vi "Actor Core.vi"(8 "error in":errorcluster, 11 "Settings Actor in":refnum<class "Settings Actor.lvclass">) -> (0 "error out":errorcluster, 3 "Actor out":refnum<class "Actor.lvclass">)   [LabVIEW 2021, in "Settings Module.lvlib" / "Settings Actor.lvclass"]
doc: "The user interface for this panel.\n\n----\nPlease see the following web address for additional documentation and tutorial information:\nhttp://www.mooregoodideas.com/mgi-panel-manager/\n\nAuthor: Derek Trepanier\n\nCopyright (c) 2018, Moore Good Ideas, Inc.\n\nAll rights reserved.\n\nRedistribution and use in source and binary forms, with or without modification, are permitted provided that the following conditions are met:\n\n * Redistributions of source code must retain the above copyright notice, this list of conditions and the following disclaimer.\n * Redistributions in binary form must reproduce the above copyright notice, this list of conditions and the following disclaimer in the documentation and/or other materials provided with the distribution.\n * Neither the name of Moore Good Ideas, Inc. nor the names of its contributors may be used to endorse or promote products derived from this software without specific prior written permission.\n\nTHIS SOFTWARE IS PROVIDED BY THE COPYRIGHT HOLDERS AND CONTRIBUTORS \"AS IS\" AND ANY EXPRESS OR IMPLIED WARRANTIES, INCLUDING, BUT NOT LIMITED TO, THE IMPLIED WARRANTIES OF MERCHANTABILITY AND FITNESS FOR A PARTICULAR PURPOSE ARE DISCLAIMED. IN NO EVENT SHALL THE COPYRIGHT OWNER OR CONTRIBUTORS BE LIABLE FOR ANY DIRECT, INDIRECT, INCIDENTAL, SPECIAL, EXEMPLARY, OR CONSEQUENTIAL DAMAGES (INCLUDING, BUT NOT LIMITED TO, PROCUREMENT OF SUBSTITUTE GOODS OR SERVICES; LOSS OF USE, DATA, OR PROFITS; OR BUSINESS INTERRUPTION) HOWEVER CAUSED AND ON ANY THEORY OF LIABILITY, WHETHER IN CONTRACT, STRICT LIABILITY, OR TORT (INCLUDING NEGLIGENCE OR OTHERWISE) ARISING IN ANY WAY OUT OF THE USE OF THIS SOFTWARE, EVEN IF ADVISED OF THE POSSIBILITY OF SUCH DAMAGE."
uses:
  Settings Actor.lvclass
  C:/Program Files (x86)/National Instruments/LabVIEW 2021/vi.lib/MGI/Panel Manager/Panel Actor/Panel Actor/Panel Actor.lvclass
  <vilib>/ActorFramework/Actor/Actor.lvclass
  <vilib>/ActorFramework/Message Enqueuer/Message Enqueuer.lvclass/Message Enqueuer.ctl
  Appearance Actor/Appearance Actor/Typedefs/User Event-Panel Resize-Data--cluster.ctl
  <vilib>/Utility/miscctls.llb/LVRectTypeDef.ctl
  <vilib>/event_ctls.llb/sizeaction.ctl
  <vilib>/event_ctls.llb/panelstate.ctl
  Appearance Actor/Appearance Actor Messages/User Event-Panel Resize Msg/User Event-Panel Resize Msg.lvclass/User Event-Panel Resize Msg.ctl
  <vilib>/ActorFramework/Message Enqueuer/Enqueue.vi
  <vilib>/ActorFramework/Stop Msg/Stop Msg.lvclass
  C:/Program Files (x86)/National Instruments/LabVIEW 2021/vi.lib/ActorFramework/Message/Message.lvclass
  Appearance Actor/Appearance Actor Messages/User Event-Title Bar-Mouse Down Msg/User Event-Title Bar-Mouse Down Msg.lvclass
  Appearance Actor/Appearance Actor Messages/User Event-Close-Value Change Msg/User Event-Close-Value Change Msg.lvclass
  Appearance Actor/Appearance Actor Messages/User Event-Maximize-Value Change Msg/User Event-Maximize-Value Change Msg.lvclass
  Appearance Actor/Appearance Actor Messages/User Event-Minimize-Value Change Msg/User Event-Minimize-Value Change Msg.lvclass
  Appearance Actor/Appearance Actor Messages/User Event-Undock-Value Change Msg/User Event-Undock-Value Change Msg.lvclass
  Appearance Actor/Appearance Actor Messages/User Event-Panel Resize Msg/User Event-Panel Resize Msg.lvclass
  <vilib>/ActorFramework/Message Priority Queue/Priority Enqueue.vi
  Appearance Actor/Appearance Actor/Appearance Actor.lvclass
  <vilib>/MGI/Panel Manager/Panel Actor/Panel Actor/Panel Actor.lvclass
  <vilib>/MGI/Panel Manager/Panel Actor/Panel Actor Messages/Show Panel Msg/Show Panel Msg.lvclass
panel:
  in  "Title Bar L":bool
  out "TB.Icon":u16(ring)
  in  "Title Bar M":bool
  out "TB.Title":string
  in  "TB.Light-Button.Undock":bool
  in  "TB.Light-CloseButton":bool
  in  "TB.Light-Button.Maximize":bool
  in  "TB.Light-Button.Minimize":bool
  in  "TB.Dark-Button.Undock":bool
  in  "TB.Dark-CloseButton":bool
  in  "TB.Dark-Button.Maximize":bool
  in  "TB.Dark-Button.Minimize":bool
  in  "Title Bar R":bool
  in  "SM.Light-RadioButton":T1(radio) caption="Radio Buttons"
  in  "SM.Dark-RadioButton":T1(radio) caption="Radio Buttons"
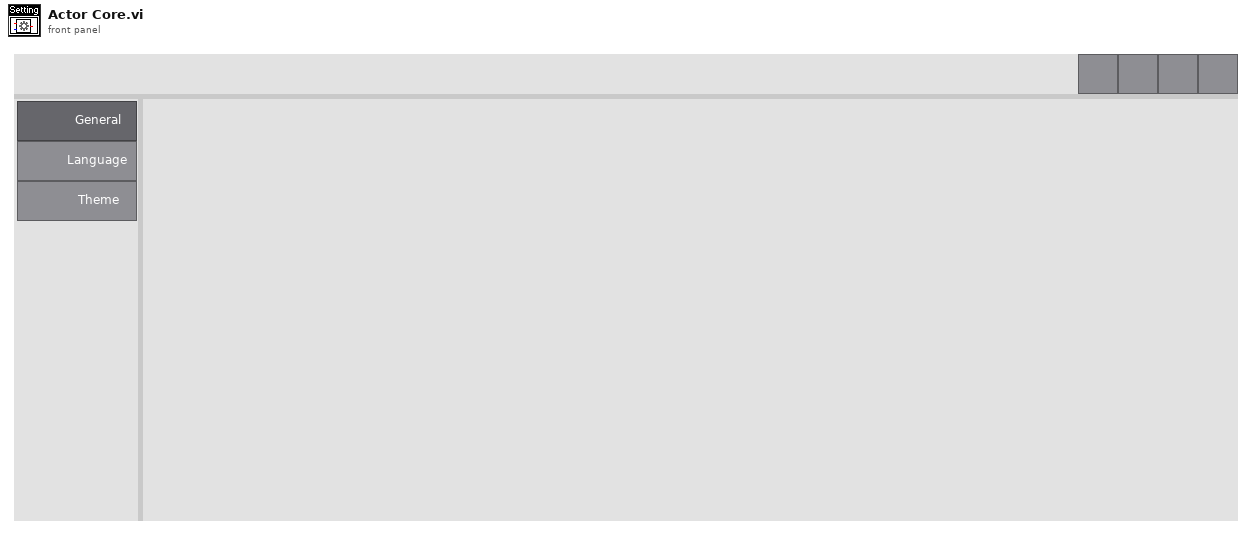
[diagram p1: front panel]
types:
  T1 = enum32{"SM.RadioButton.General", "SM.RadioButton.Language", "SM.RadioButton.Theme"}
  T2 = typedef "Appearance Actor.lvlib/Appearance Actor.lvclass/User Event-Panel Resize-Data--cluster.ctl" = cluster{"OldBnds":T3, "NewBnds":T3, "Act":T4, "PrevState":T5}
  T3 = typedef "LVRectTypeDef.ctl" = cluster{"Left":i16, "Top":i16, "Right":i16, "Bottom":i16}
  T4 = typedef "sizeaction.ctl" = enum32{"Minimized", "Maximized", "Resized"}
  T5 = typedef "panelstate.ctl" = enum32{"Standard", "Minimized", "Maximized"}
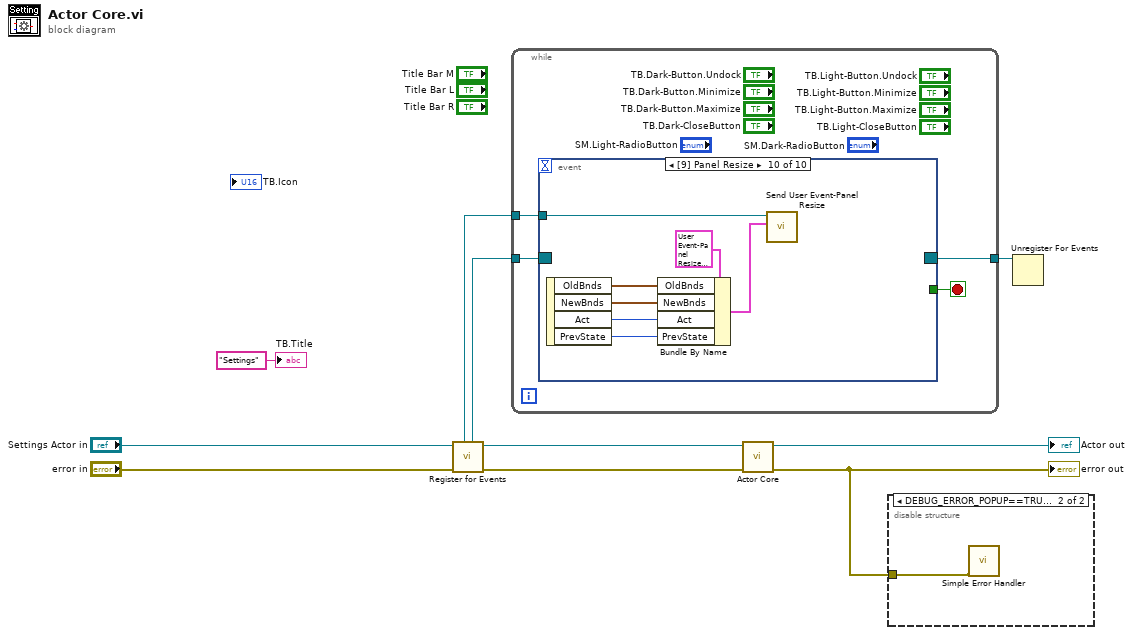
[diagram p0: block diagram]
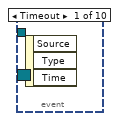
[diagram p3: hidden frame]
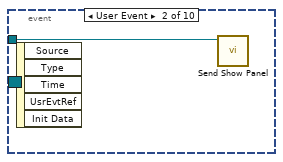
[diagram p4: hidden frame]
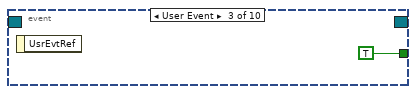
[diagram p5: hidden frame]
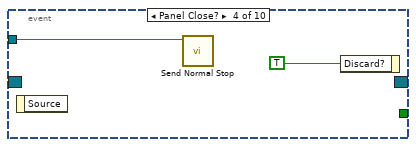
[diagram p6: hidden frame]
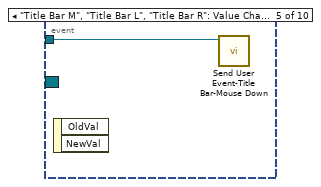
[diagram p7: hidden frame]
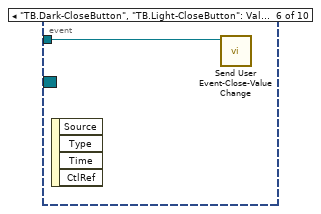
[diagram p8: hidden frame]
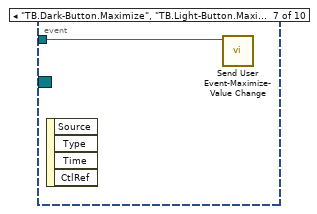
[diagram p9: hidden frame]
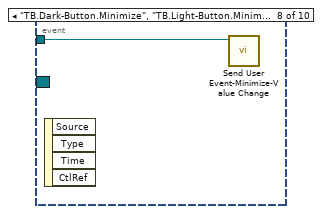
[diagram p10: hidden frame]
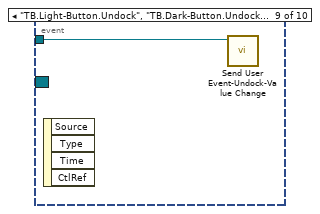
[diagram p11: hidden frame]
diagram:
  n1 = call <vilib>:"Register for Events.vi"("Error In"="error in", "Panel Actor in"="Settings Actor in") -> ("Error Out"=w6:errorcluster, "Panel Actor out"=w4:refnum<class "Settings Actor.lvclass">, "Pnl Actor"=w2:refnum<event-registration>, "Self Enqueuer"=w3:refnum<class "Message Enqueuer.lvclass">)  [unwired: 6 in]
  n2 = while {
    tunnel: w2 -> [w14]
    tunnel: w3 -> [w13]
    tunnel: [w11] -> w7
    stop <- w12 stop-if-true
    n3 = event shown="[9] Panel Resize" {
      selector: w14 -> [_ _ _ _ _ _ _ _ _ _]
      dyn-events: [_ _ _ _ _ _ _ _ _ _] -> w11
      timeout: _ -> [_ _ _ _ _ _ _ _ _ _]
      tunnel: w13 -> [_ w15 _ w18 w19 w20 w21 w22 w23 w30]
      tunnel: [_ _ TRUE _ _ _ _ _ _ _] -> w12
      event Timeout {
        n4 = event-data() -> ()  [unwired: 1 in, 3 out]
      }
      event User Event {
        n5 = event-data() -> ()  [unwired: 1 in, 5 out]
        n6 = call <vilib>:"Send Show Panel.vi"("Message Enqueuer in"=w15) -> ()  [unwired: 9 in, 2 out]
      }
      event User Event {
        n7 = event-data() -> ()  [unwired: 1 in, 1 out]
      }
      event Panel Close? {
        n8 = event-data() -> ()  [unwired: 1 in, 1 out]
        n9 = call <vilib>:"Send Normal Stop.vi"("Message Enqueuer"=w18) -> ()  [unwired: 10 in, 1 out]
        n10 = event-data("Discard?"=TRUE) -> ()  [unwired: 1 in, 1 out]
      }
      event "Title Bar M", "Title Bar L", "Title Bar R": Value Change {
        n11 = event-data() -> ()  [unwired: 1 in, 2 out]
        n12 = call "Send User Event-Title Bar-Mouse Down.vi"("Message Enqueuer"=w19) -> ()  [unwired: 9 in, 2 out]
      }
      event "TB.Dark-CloseButton", "TB.Light-CloseButton": Value Change {
        n13 = event-data() -> ()  [unwired: 1 in, 4 out]
        n14 = call "Send User Event-Close-Value Change.vi"("Message Enqueuer"=w20) -> ()  [unwired: 9 in, 2 out]
      }
      event "TB.Dark-Button.Maximize", "TB.Light-Button.Maximize": Value Change {
        n15 = event-data() -> ()  [unwired: 1 in, 4 out]
        n16 = call "Send User Event-Maximize-Value Change.vi"("Message Enqueuer"=w21) -> ()  [unwired: 9 in, 2 out]
      }
      event "TB.Dark-Button.Minimize", "TB.Light-Button.Minimize": Value Change {
        n17 = event-data() -> ()  [unwired: 1 in, 4 out]
        n18 = call "Send User Event-Minimize-Value Change.vi"("Message Enqueuer"=w22) -> ()  [unwired: 9 in, 2 out]
      }
      event "TB.Light-Button.Undock", "TB.Dark-Button.Undock": Value Change {
        n19 = event-data() -> ()  [unwired: 1 in, 4 out]
        n20 = call "Send User Event-Undock-Value Change.vi"("Message Enqueuer"=w23) -> ()  [unwired: 9 in, 2 out]
      }
      event Panel Resize {
        n21 = event-data() -> ("OldBnds"=w29:T3, "NewBnds"=w26:T3, "Act"=w27:T4, "PrevState"=w28:T5)  [unwired: 1 in]
        n22 = Bundle By Name(cluster=T2 {"OldBnds"={"Left"=0, "Top"=0, "Right"=0, "Bottom"=0}, "NewBnds"={"Left"=0, "Top"=0, "Right"=0, "Bottom"=0}, "Act"=enum."Resized", "PrevState"=enum."Standard"} ("Panel Resize Data"), "OldBnds"=w29, "NewBnds"=w26, "Act"=w27, "PrevState"=w28) -> (w25:T2)
        n23 = call "Send User Event-Panel Resize.vi"("Panel Resize Data"=w25, "Message Enqueuer"=w30) -> ()  [unwired: 8 in, 2 out]
      }
    }
  }
  n24 = call-parent "Actor Core.vi"("error in"=w6, "Appearance Actor in"=w4) -> ("error out"=w1:errorcluster, "Actor out"=→"Actor out":refnum<class "Actor.lvclass">)  [unwired: 8 in]
  "error out" <- w1
  n25 = disable-structure shown="DEBUG_ERROR_POPUP==TRUE" {
    disable-tunnel: w1 -> [_ w31]
    frame condition #0 {
    }
    frame condition #1 (active) {
      n26 = call <vilib>:"Simple Error Handler.vi"("error in (no error)"=w31) -> ()  [unwired: 4 in, 5 out]
    }
  }
  n27 = Unregister For Events(event registration refnum=w7) -> ()  [unwired: 1 in, 1 out]
  "TB.Title" <- "Settings" ("TB.Title")
